vi "FipsAdjacent.vi"() -> (11 "Fips":i32[](array[numeric]))   [LabVIEW 2017] (continued)
MO\"\t29205\t\"Knox County, MO\"\t29103\n\"Shelby County, MO\"\t29205\t\"Lewis County, MO\"\t29111\n\"Shelby County, MO\"\t29205\t\"Macon County, MO\"\t29121\n\"Shelby County, MO\"\t29205\t\"Marion County, MO\"\t29127\n\"Shelby County, MO\"\t29205\t\"Monroe County, MO\"\t29137\n\"Shelby County, MO\"\t29205\t\"Shelby County, MO\"\t29205\n\"Stoddard County, MO\"\t29207\t\"Bollinger County, MO\"\t29017\n\"Stoddard County, MO\"\t29207\t\"Butler County, MO\"\t29023\n\"Stoddard County, MO\"\t29207\t\"Cape Girardeau County, MO\"\t29031\n\"Stoddard County, MO\"\t29207\t\"Dunklin County, MO\"\t29069\n\"Stoddard County, MO\"\t29207\t\"New Madrid County, MO\"\t29143\n\"Stoddard County, MO\"\t29207\t\"Scott County, MO\"\t29201\n\"Stoddard County, MO\"\t29207\t\"Stoddard County, MO\"\t29207\n\"Stoddard County, MO\"\t29207\t\"Wayne County, MO\"\t29223\n\"Stone County, MO\"\t29209\t\"Carroll County, AR\"\t05015\n\"Stone County, MO\"\t29209\t\"Barry County, MO\"\t29009\n\"Stone County, MO\"\t29209\t\"Christian County, MO\"\t29043\n\"Stone County, MO\"\t29209\t\"Lawrence County, MO\"\t29109\n\"Stone County, MO\"\t29209\t\"Stone County, MO\"\t29209\n\"Stone County, MO\"\t29209\t\"Taney County, MO\"\t29213\n\"Sullivan County, MO\"\t29211\t\"Adair County, MO\"\t29001\n\"Sullivan County, MO\"\t29211\t\"Grundy County, MO\"\t29079\n\"Sullivan County, MO\"\t29211\t\"Linn County, MO\"\t29115\n\"Sullivan County, MO\"\t29211\t\"Mercer County, MO\"\t29129\n\"Sullivan County, MO\"\t29211\t\"Putnam County, MO\"\t29171\n\"Sullivan County, MO\"\t29211\t\"Sullivan County, MO\"\t29211\n\"Taney County, MO\"\t29213\t\"Boone County, AR\"\t05009\n\"Taney County, MO\"\t29213\t\"Carroll County, AR\"\t05015\n\"Taney County, MO\"\t29213\t\"Marion County, AR\"\t05089\n\"Taney County, MO\"\t29213\t\"Christian County, MO\"\t29043\n\"Taney County, MO\"\t29213\t\"Douglas County, MO\"\t29067\n\"Taney County, MO\"\t29213\t\"Ozark County, MO\"\t29153\n\"Taney County, MO\"\t29213\t\"Stone County, MO\"\t29209\n\"Taney County, MO\"\t29213\t\"Taney County, MO\"\t29213\n\"Texas County, MO\"\t29215\t\"Dent County, MO\"\t29065\n\"Texas County, MO\"\t29215\t\"Douglas County, MO\"\t29067\n\"Texas County, MO\"\t29215\t\"Howell County, MO\"\t29091\n\"Texas County, MO\"\t29215\t\"Laclede County, MO\"\t29105\n\"Texas County, MO\"\t29215\t\"Phelps County, MO\"\t29161\n\"Texas County, MO\"\t29215\t\"Pulaski County, MO\"\t29169\n\"Texas County, MO\"\t29215\t\"Shannon County, MO\"\t29203\n\"Texas County, MO\"\t29215\t\"Texas County, MO\"\t29215\n\"Texas County, MO\"\t29215\t\"Wright County, MO\"\t29229\n\"Vernon County, MO\"\t29217\t\"Bourbon County, KS\"\t20011\n\"Vernon County, MO\"\t29217\t\"Crawford County, KS\"\t20037\n\"Vernon County, MO\"\t29217\t\"Linn County, KS\"\t20107\n\"Vernon County, MO\"\t29217\t\"Barton County, MO\"\t29011\n\"Vernon County, MO\"\t29217\t\"Bates County, MO\"\t29013\n\"Vernon County, MO\"\t29217\t\"Cedar County, MO\"\t29039\n\"Vernon County, MO\"\t29217\t\"St. Clair County, MO\"\t29185\n\"Vernon County, MO\"\t29217\t\"Vernon County, MO\"\t29217\n\"Warren County, MO\"\t29219\t\"Franklin County, MO\"\t29071\n\"Warren County, MO\"\t29219\t\"Gasconade County, MO\"\t29073\n\"Warren County, MO\"\t29219\t\"Lincoln County, MO\"\t29113\n\"Warren County, MO\"\t29219\t\"Montgomery County, MO\"\t29139\n\"Warren County, MO\"\t29219\t\"St. Charles County, MO\"\t29183\n\"Warren County, MO\"\t29219\t\"Warren County, MO\"\t29219\n\"Washington County, MO\"\t29221\t\"Crawford County, MO\"\t29055\n\"Washington County, MO\"\t29221\t\"Franklin County, MO\"\t29071\n\"Washington County, MO\"\t29221\t\"Iron County, MO\"\t29093\n\"Washington County, MO\"\t29221\t\"Jefferson County, MO\"\t29099\n\"Washington County, MO\"\t29221\t\"St. Francois County, MO\"\t29187\n\"Washington County, MO\"\t29221\t\"Washington County, MO\"\t29221\n\"Wayne County, MO\"\t29223\t\"Bollinger County, MO\"\t29017\n\"Wayne County, MO\"\t29223\t\"Butler County, MO\"\t29023\n\"Wayne County, MO\"\t29223\t\"Carter County, MO\"\t29035\n\"Wayne County, MO\"\t29223\t\"Iron County, MO\"\t29093\n\"Wayne County, MO\"\t29223\t\"Madison County, MO\"\t29123\n\"Wayne County, MO\"\t29223\t\"Reynolds County, MO\"\t29179\n\"Wayne County, MO\"\t29223\t\"Stoddard County, MO\"\t29207\n\"Wayne County, MO\"\t29223\t\"Wayne County, MO\"\t29223\n\"Webster County, MO\"\t29225\t\"Christian County, MO\"\t29043\n\"Webster County, MO\"\t29225\t\"Dallas County, MO\"\t29059\n\"Webster County, MO\"\t29225\t\"Douglas County, MO\"\t29067\n\"Webster County, MO\"\t29225\t\"Greene County, MO\"\t29077\n\"Webster County, MO\"\t29225\t\"Laclede County, MO\"\t29105\n\"Webster County, MO\"\t29225\t\"Webster County, MO\"\t29225\n\"Webster County, MO\"\t29225\t\"Wright County, MO\"\t29229\n\"Worth County, MO\"\t29227\t\"Ringgold County, IA\"\t19159\n\"Worth County, MO\"\t29227\t\"Taylor County, IA\"\t19173\n\"Worth County, MO\"\t29227\t\"Gentry County, MO\"\t29075\n\"Worth County, MO\"\t29227\t\"Harrison County, MO\"\t29081\n\"Worth County, MO\"\t29227\t\"Nodaway County, MO\"\t29147\n\"Worth County, MO\"\t29227\t\"Worth County, MO\"\t29227\n\"Wright County, MO\"\t29229\t\"Douglas County, MO\"\t29067\n\"Wright County, MO\"\t29229\t\"Laclede County, MO\"\t29105\n\"Wright County, MO\"\t29229\t\"Texas County, MO\"\t29215\n\"Wright County, MO\"\t29229\t\"Webster County, MO\"\t29225\n\"Wright County, MO\"\t29229\t\"Wright County, MO\"\t29229\n\"St. Louis city, MO\"\t29510\t\"Madison County, IL\"\t17119\n\"St. Louis city, MO\"\t29510\t\"St. Clair County, IL\"\t17163\n\"St. Louis city, MO\"\t29510\t\"St. Louis County, MO\"\t29189\n\"St. Louis city, MO\"\t29510\t\"St. Louis city, MO\"\t29510\n\"Beaverhead County, MT\"\t30001\t\"Clark County, ID\"\t16033\n\"Beaverhead County, MT\"\t30001\t\"Fremont County, ID\"\t16043\n\"Beaverhead County, MT\"\t30001\t\"Lemhi County, ID\"\t16059\n\"Beaverhead County, MT\"\t30001\t\"Beaverhead County, MT\"\t30001\n\"Beaverhead County, MT\"\t30001\t\"Deer Lodge County, MT\"\t30023\n\"Beaverhead County, MT\"\t30001\t\"Madison County, MT\"\t30057\n\"Beaverhead County, MT\"\t30001\t\"Ravalli County, MT\"\t30081\n\"Beaverhead County, MT\"\t30001\t\"Silver Bow County, MT\"\t30093\n\"Big Horn County, MT\"\t30003\t\"Big Horn County, MT\"\t30003\n\"Big Horn County, MT\"\t30003\t\"Carbon County, MT\"\t30009\n\"Big Horn County, MT\"\t30003\t\"Powder River County, MT\"\t30075\n\"Big Horn County, MT\"\t30003\t\"Rosebud County, MT\"\t30087\n\"Big Horn County, MT\"\t30003\t\"Treasure County, MT\"\t30103\n\"Big Horn County, MT\"\t30003\t\"Yellowstone County, MT\"\t30111\n\"Big Horn County, MT\"\t30003\t\"Big Horn County, WY\"\t56003\n\"Big Horn County, MT\"\t30003\t\"Sheridan County, WY\"\t56033\n\"Blaine County, MT\"\t30005\t\"Blaine County, MT\"\t30005\n\"Blaine County, MT\"\t30005\t\"Chouteau County, MT\"\t30015\n\"Blaine County, MT\"\t30005\t\"Fergus County, MT\"\t30027\n\"Blaine County, MT\"\t30005\t\"Hill County, MT\"\t30041\n\"Blaine County, MT\"\t30005\t\"Phillips County, MT\"\t30071\n\"Broadwater County, MT\"\t30007\t\"Broadwater County, MT\"\t30007\n\"Broadwater County, MT\"\t30007\t\"Gallatin County, MT\"\t30031\n\"Broadwater County, MT\"\t30007\t\"Jefferson County, MT\"\t30043\n\"Broadwater County, MT\"\t30007\t\"Lewis and Clark County, MT\"\t30049\n\"Broadwater County, MT\"\t30007\t\"Meagher County, MT\"\t30059\n\"Carbon County, MT\"\t30009\t\"Big Horn County, MT\"\t30003\n\"Carbon County, MT\"\t30009\t\"Carbon County, MT\"\t30009\n\"Carbon County, MT\"\t30009\t\"Park County, MT\"\t30067\n\"Carbon County, MT\"\t30009\t\"Stillwater County, MT\"\t30095\n\"Carbon County, MT\"\t30009\t\"Yellowstone County, MT\"\t30111\n\"Carbon County, MT\"\t30009\t\"Big Horn County, WY\"\t56003\n\"Carbon County, MT\"\t30009\t\"Park County, WY\"\t56029\n\"Carter County, MT\"\t30011\t\"Carter County, MT\"\t30011\n\"Carter County, MT\"\t30011\t\"Custer County, MT\"\t30017\n\"Carter County, MT\"\t30011\t\"Fallon County, MT\"\t30025\n\"Carter County, MT\"\t30011\t\"Powder River County, MT\"\t30075\n\"Carter County, MT\"\t30011\t\"Butte County, SD\"\t46019\n\"Carter County, MT\"\t30011\t\"Harding County, SD\"\t46063\n\"Carter County, MT\"\t30011\t\"Crook County, WY\"\t56011\n\"Cascade County, MT\"\t30013\t\"Cascade County, MT\"\t30013\n\"Cascade County, MT\"\t30013\t\"Chouteau County, MT\"\t30015\n\"Cascade County, MT\"\t30013\t\"Judith Basin County, MT\"\t30045\n\"Cascade County, MT\"\t30013\t\"Lewis and Clark County, MT\"\t30049\n\"Cascade County, MT\"\t30013\t\"Meagher County, MT\"\t30059\n\"Cascade County, MT\"\t30013\t\"Teton County, MT\"\t30099\n\"Chouteau County, MT\"\t30015\t\"Blaine County, MT\"\t30005\n\"Chouteau County, MT\"\t30015\t\"Cascade County, MT\"\t30013\n\"Chouteau County, MT\"\t30015\t\"Chouteau County, MT\"\t30015\n\"Chouteau County, MT\"\t30015\t\"Fergus County, MT\"\t30027\n\"Chouteau County, MT\"\t30015\t\"Hill County, MT\"\t30041\n\"Chouteau County, MT\"\t30015\t\"Judith Basin County, MT\"\t30045\n\"Chouteau County, MT\"\t30015\t\"Liberty County, MT\"\t30051\n\"Chouteau County, MT\"\t30015\t\"Pondera County, MT\"\t30073\n\"Chouteau County, MT\"\t30015\t\"Teton County, MT\"\t30099\n\"Custer County, MT\"\t30017\t\"Carter County, MT\"\t30011\n\"Custer County, MT\"\t30017\t\"Custer County, MT\"\t30017\n\"Custer County, MT\"\t30017\t\"Fallon County, MT\"\t30025\n\"Custer County, MT\"\t30017\t\"Garfield County, MT\"\t30033\n\"Custer County, MT\"\t30017\t\"Powder River County, MT\"\t30075\n\"Custer County, MT\"\t30017\t\"Prairie County, MT\"\t30079\n\"Custer County, MT\"\t30017\t\"Rosebud County, MT\"\t30087\n\"Daniels County, MT\"\t30019\t\"Daniels County, MT\"\t30019\n\"Daniels County, MT\"\t30019\t\"Roosevelt County, MT\"\t30085\n\"Daniels County, MT\"\t30019\t\"Sheridan County, MT\"\t30091\n\"Daniels County, MT\"\t30019\t\"Valley County, MT\"\t30105\n\"Dawson County, MT\"\t30021\t\"Dawson County, MT\"\t30021\n\"Dawson County, MT\"\t30021\t\"McCone County, MT\"\t30055\n\"Dawson County, MT\"\t30021\t\"Prairie County, MT\"\t30079\n\"Dawson County, MT\"\t30021\t\"Richland County, MT\"\t30083\n\"Dawson County, MT\"\t30021\t\"Wibaux County, MT\"\t30109\n\"Deer Lodge County, MT\"\t30023\t\"Beaverhead County, MT\"\t30001\n\"Deer Lodge County, MT\"\t30023\t\"Deer Lodge County, MT\"\t30023\n\"Deer Lodge County, MT\"\t30023\t\"Granite County, MT\"\t30039\n\"Deer Lodge County, MT\"\t30023\t\"Jefferson County, MT\"\t30043\n\"Deer Lodge County, MT\"\t30023\t\"Powell County, MT\"\t30077\n\"Deer Lodge County, MT\"\t30023\t\"Ravalli County, MT\"\t30081\n\"Deer Lodge County, MT\"\t30023\t\"Silver Bow County, MT\"\t30093\n\"Fallon County, MT\"\t30025\t\"Carter County, MT\"\t30011\n\"Fallon County, MT\"\t30025\t\"Custer County, MT\"\t30017\n\"Fallon County, MT\"\t30025\t\"Fallon County, MT\"\t30025\n\"Fallon County, MT\"\t30025\t\"Prairie County, MT\"\t30079\n\"Fallon County, MT\"\t30025\t\"Wibaux County, MT\"\t30109\n\"Fallon County, MT\"\t30025\t\"Bowman County, ND\"\t38011\n\"Fallon County, MT\"\t30025\t\"Golden Valley County, ND\"\t38033\n\"Fallon County, MT\"\t30025\t\"Slope County, ND\"\t38087\n\"Fallon County, MT\"\t30025\t\"Harding County, SD\"\t46063\n\"Fergus County, MT\"\t30027\t\"Blaine County, MT\"\t30005\n\"Fergus County, MT\"\t30027\t\"Chouteau County, MT\"\t30015\n\"Fergus County, MT\"\t30027\t\"Fergus County, MT\"\t30027\n\"Fergus County, MT\"\t30027\t\"Golden Valley County, MT\"\t30037\n\"Fergus County, MT\"\t30027\t\"Judith Basin County, MT\"\t30045\n\"Fergus County, MT\"\t30027\t\"Musselshell County, MT\"\t30065\n\"Fergus County, MT\"\t30027\t\"Petroleum County, MT\"\t30069\n\"Fergus County, MT\"\t30027\t\"Phillips County, MT\"\t30071\n\"Fergus County, MT\"\t30027\t\"Wheatland County, MT\"\t30107\n\"Flathead County, MT\"\t30029\t\"Flathead County, MT\"\t30029\n\"Flathead County, MT\"\t30029\t\"Glacier County, MT\"\t30035\n\"Flathead County, MT\"\t30029\t\"Lake County, MT\"\t30047\n\"Flathead County, MT\"\t30029\t\"Lewis and Clark County, MT\"\t30049\n\"Flathead County, MT\"\t30029\t\"Lincoln County, MT\"\t30053\n\"Flathead County, MT\"\t30029\t\"Missoula County, MT\"\t30063\n\"Flathead County, MT\"\t30029\t\"Pondera County, MT\"\t30073\n\"Flathead County, MT\"\t30029\t\"Powell County, MT\"\t30077\n\"Flathead County, MT\"\t30029\t\"Sanders County, MT\"\t30089\n\"Flathead County, MT\"\t30029\t\"Teton County, MT\"\t30099\n\"Gallatin County, MT\"\t30031\t\"Fremont County, ID\"\t16043\n\"Gallatin County, MT\"\t30031\t\"Broadwater County, MT\"\t30007\n\"Gallatin County, MT\"\t30031\t\"Gallatin County, MT\"\t30031\n\"Gallatin County, MT\"\t30031\t\"Jefferson County, MT\"\t30043\n\"Gallatin County, MT\"\t30031\t\"Madison County, MT\"\t30057\n\"Gallatin County, MT\"\t30031\t\"Meagher County, MT\"\t30059\n\"Gallatin County, MT\"\t30031\t\"Park County, MT\"\t30067\n\"Gallatin County, MT\"\t30031\t\"Park County, WY\"\t56029\n\"Gallatin County, MT\"\t30031\t\"Teton County, WY\"\t56039\n\"Garfield County, MT\"\t30033\t\"Custer County, MT\"\t30017\n\"Garfield County, MT\"\t30033\t\"Garfield County, MT\"\t30033\n\"Garfield County, MT\"\t30033\t\"McCone County, MT\"\t30055\n\"Garfield County, MT\"\t30033\t\"Petroleum County, MT\"\t30069\n\"Garfield County, MT\"\t30033\t\"Phillips County, MT\"\t30071\n\"Garfield County, MT\"\t30033\t\"Prairie County, MT\"\t30079\n\"Garfield County, MT\"\t30033\t\"Rosebud County, MT\"\t30087\n\"Garfield County, MT\"\t30033\t\"Valley County, MT\"\t30105\n\"Glacier County, MT\"\t30035\t\"Flathead County, MT\"\t30029\n\"Glacier County, MT\"\t30035\t\"Glacier County, MT\"\t30035\n\"Glacier County, MT\"\t30035\t\"Pondera County, MT\"\t30073\n\"Glacier County, MT\"\t30035\t\"Toole County, MT\"\t30101\n\"Golden Valley County, MT\"\t30037\t\"Fergus County, MT\"\t30027\n\"Golden Valley County, MT\"\t30037\t\"Golden Valley County, MT\"\t30037\n\"Golden Valley County, MT\"\t30037\t\"Musselshell County, MT\"\t30065\n\"Golden Valley County, MT\"\t30037\t\"Stillwater County, MT\"\t30095\n\"Golden Valley County, MT\"\t30037\t\"Sweet Grass County, MT\"\t30097\n\"Golden Valley County, MT\"\t30037\t\"Wheatland County, MT\"\t30107\n\"Golden Valley County, MT\"\t30037\t\"Yellowstone County, MT\"\t30111\n\"Granite County, MT\"\t30039\t\"Deer Lodge County, MT\"\t30023\n\"Granite County, MT\"\t30039\t\"Granite County, MT\"\t30039\n\"Granite County, MT\"\t30039\t\"Missoula County, MT\"\t30063\n\"Granite County, MT\"\t30039\t\"Powell County, MT\"\t30077\n\"Granite County, MT\"\t30039\t\"Ravalli County, MT\"\t30081\n\"Hill County, MT\"\t30041\t\"Blaine County, MT\"\t30005\n\"Hill County, MT\"\t30041\t\"Chouteau County, MT\"\t30015\n\"Hill County, MT\"\t30041\t\"Hill County, MT\"\t30041\n\"Hill County, MT\"\t30041\t\"Liberty County, MT\"\t30051\n\"Jefferson County, MT\"\t30043\t\"Broadwater County, MT\"\t30007\n\"Jefferson County, MT\"\t30043\t\"Deer Lodge County, MT\"\t30023\n\"Jefferson County, MT\"\t30043\t\"Gallatin County, MT\"\t30031\n\"Jefferson County, MT\"\t30043\t\"Jefferson County, MT\"\t30043\n\"Jefferson County, MT\"\t30043\t\"Lewis and Clark County, MT\"\t30049\n\"Jefferson County, MT\"\t30043\t\"Madison County, MT\"\t30057\n\"Jefferson County, MT\"\t30043\t\"Powell County, MT\"\t30077\n\"Jefferson County, MT\"\t30043\t\"Silver Bow County, MT\"\t30093\n\"Judith Basin County, MT\"\t30045\t\"Cascade County, MT\"\t30013\n\"Judith Basin County, MT\"\t30045\t\"Chouteau County, MT\"\t30015\n\"Judith Basin County, MT\"\t30045\t\"Fergus County, MT\"\t30027\n\"Judith Basin County, MT\"\t30045\t\"Judith Basin County, MT\"\t30045\n\"Judith Basin County, MT\"\t30045\t\"Meagher County, MT\"\t30059\n\"Judith Basin County, MT\"\t30045\t\"Wheatland County, MT\"\t30107\n\"Lake County, MT\"\t30047\t\"Flathead County, MT\"\t30029\n\"Lake County, MT\"\t30047\t\"Lake County, MT\"\t30047\n\"Lake County, MT\"\t30047\t\"Missoula County, MT\"\t30063\n\"Lake County, MT\"\t30047\t\"Sanders County, MT\"\t30089\n\"Lewis and Clark County, MT\"\t30049\t\"Broadwater County, MT\"\t30007\n\"Lewis and Clark County, MT\"\t30049\t\"Cascade County, MT\"\t30013\n\"Lewis and Clark County, MT\"\t30049\t\"Flathead County, MT\"\t30029\n\"Lewis and Clark County, MT\"\t30049\t\"Jefferson County, MT\"\t30043\n\"Lewis and Clark County, MT\"\t30049\t\"Lewis and Clark County, MT\"\t30049\n\"Lewis and Clark County, MT\"\t30049\t\"Meagher County, MT\"\t30059\n\"Lewis and Clark County, MT\"\t30049\t\"Powell County, MT\"\t30077\n\"Lewis and Clark County, MT\"\t30049\t\"Teton County, MT\"\t30099\n\"Liberty County, MT\"\t30051\t\"Chouteau County, MT\"\t30015\n\"Liberty County, MT\"\t30051\t\"Hill County, MT\"\t30041\n\"Liberty County, MT\"\t30051\t\"Liberty County, MT\"\t30051\n\"Liberty County, MT\"\t30051\t\"Pondera County, MT\"\t30073\n\"Liberty County, MT\"\t30051\t\"Toole County, MT\"\t30101\n\"Lincoln County, MT\"\t30053\t\"Bonner County, ID\"\t16017\n\"Lincoln County, MT\"\t30053\t\"Boundary County, ID\"\t16021\n\"Lincoln County, MT\"\t30053\t\"Flathead County, MT\"\t30029\n\"Lincoln County, MT\"\t30053\t\"Lincoln County, MT\"\t30053\n\"Lincoln County, MT\"\t30053\t\"Sanders County, MT\"\t30089\n\"McCone County, MT\"\t30055\t\"Dawson County, MT\"\t30021\n\"McCone County, MT\"\t30055\t\"Garfield County, MT\"\t30033\n\"McCone County, MT\"\t30055\t\"McCone County, MT\"\t30055\n\"McCone County, MT\"\t30055\t\"Prairie County, MT\"\t30079\n\"McCone County, MT\"\t30055\t\"Richland County, MT\"\t30083\n\"McCone County, MT\"\t30055\t\"Roosevelt County, MT\"\t30085\n\"McCone County, MT\"\t30055\t\"Valley County, MT\"\t30105\n\"Madison County, MT\"\t30057\t\"Fremont County, ID\"\t16043\n\"Madison County, MT\"\t30057\t\"Beaverhead County, MT\"\t30001\n\"Madison County, MT\"\t30057\t\"Gallatin County, MT\"\t30031\n\"Madison County, MT\"\t30057\t\"Jefferson County, MT\"\t30043\n\"Madison County, MT\"\t30057\t\"Madison County, MT\"\t30057\n\"Madison County, MT\"\t30057\t\"Silver Bow County, MT\"\t30093\n\"Meagher County, MT\"\t30059\t\"Broadwater County, MT\"\t30007\n\"Meagher County, MT\"\t30059\t\"Cascade County, MT\"\t30013\n\"Meagher County, MT\"\t30059\t\"Gallatin County, MT\"\t30031\n\"Meagher County, MT\"\t30059\t\"Judith Basin County, MT\"\t30045\n\"Meagher County, MT\"\t30059\t\"Lewis and Clark County, MT\"\t30049\n\"Meagher County, MT\"\t30059\t\"Meagher County, MT\"\t30059\n\"Meagher County, MT\"\t30059\t\"Park County, MT\"\t30067\n\"Meagher County, MT\"\t30059\t\"Sweet Grass County, MT\"\t30097\n\"Meagher County, MT\"\t30059\t\"Wheatland County, MT\"\t30107\n\"Mineral County, MT\"\t30061\t\"Clearwater County, ID\"\t16035\n\"Mineral County, MT\"\t30061\t\"Shoshone County, ID\"\t16079\n\"Mineral County, MT\"\t30061\t\"Mineral County, MT\"\t30061\n\"Mineral County, MT\"\t30061\t\"Missoula County, MT\"\t30063\n\"Mineral County, MT\"\t30061\t\"Sanders County, MT\"\t30089\n\"Missoula County, MT\"\t30063\t\"Clearwater County, ID\"\t16035\n\"Missoula County, MT\"\t30063\t\"Idaho County, ID\"\t16049\n\"Missoula County, MT\"\t30063\t\"Flathead County, MT\"\t30029\n\"Missoula County, MT\"\t30063\t\"Granite County, MT\"\t30039\n\"Missoula County, MT\"\t30063\t\"Lake County, MT\"\t30047\n\"Missoula County, MT\"\t30063\t\"Mineral County, MT\"\t30061\n\"Missoula County, MT\"\t30063\t\"Missoula County, MT\"\t30063\n\"Missoula County, MT\"\t30063\t\"Powell County, MT\"\t30077\n\"Missoula County, MT\"\t30063\t\"Ravalli County, MT\"\t30081\n\"Missoula County, MT\"\t30063\t\"Sanders County, MT\"\t30089\n\"Musselshell County, MT\"\t30065\t\"Fergus County, MT\"\t30027\n\"Musselshell County, MT\"\t30065\t\"Golden Valley County, MT\"\t30037\n\"Musselshell County, MT\"\t30065\t\"Musselshell County, MT\"\t30065\n\"Musselshell County, MT\"\t30065\t\"Petroleum County, MT\"\t30069\n\"Musselshell County, MT\"\t30065\t\"Rosebud County, MT\"\t30087\n\"Musselshell County, MT\"\t30065\t\"Yellowstone County, MT\"\t30111\n\"Park County, MT\"\t30067\t\"Carbon County, MT\"\t30009\n\"Park County, MT\"\t30067\t\"Gallatin County, MT\"\t30031\n\"Park County, MT\"\t30067\t\"Meagher County, MT\"\t30059\n\"Park County, MT\"\t30067\t\"Park County, MT\"\t30067\n\"Park County, MT\"\t30067\t\"Stillwater County, MT\"\t30095\n\"Park County, MT\"\t30067\t\"Sweet Grass County, MT\"\t30097\n\"Park County, MT\"\t30067\t\"Park County, WY\"\t56029\n\"Petroleum County, MT\"\t30069\t\"Fergus County, MT\"\t30027\n\"Petroleum County, MT\"\t30069\t\"Garfield County, MT\"\t30033\n\"Petroleum County, MT\"\t30069\t\"Musselshell County, MT\"\t30065\n\"Petroleum County, MT\"\t30069\t\"Petroleum County, MT\"\t30069\n\"Petroleum County, MT\"\t30069\t\"Phillips County, MT\"\t30071\n\"Petroleum County, MT\"\t30069\t\"Rosebud County, MT\"\t30087\n\"Phillips County, MT\"\t30071\t\"Blaine County, MT\"\t30005\n\"Phillips County, MT\"\t30071\t\"Fergus County, MT\"\t30027\n\"Phillips County, MT\"\t30071\t\"Garfield County, MT\"\t30033\n\"Phillips County, MT\"\t30071\t\"Petroleum County, MT\"\t30069\n\"Phillips County, MT\"\t30071\t\"Phillips County, MT\"\t30071\n\"Phillips County, MT\"\t30071\t\"Valley County, MT\"\t30105\n\"Pondera County, MT\"\t30073\t\"Chouteau County, MT\"\t30015\n\"Pondera County, MT\"\t30073\t\"Flathead County, MT\"\t30029\n\"Pondera County, MT\"\t30073\t\"Glacier County, MT\"\t30035\n\"Pondera County, MT\"\t30073\t\"Liberty County, MT\"\t30051\n\"Pondera County, MT\"\t30073\t\"Pondera County, MT\"\t30073\n\"Pondera County, MT\"\t30073\t\"Teton County, MT\"\t30099\n\"Pondera County, MT\"\t30073\t\"Toole County, MT\"\t30101\n\"Powder River County, MT\"\t30075\t\"Big Horn County, MT\"\t30003\n\"Powder River County, MT\"\t30075\t\"Carter County, MT\"\t30011\n\"Powder River County, MT\"\t30075\t\"Custer County, MT\"\t30017\n\"Powder River County, MT\"\t30075\t\"Powder River County, MT\"\t30075\n\"Powder River County, MT\"\t30075\t\"Rosebud County, MT\"\t30087\n\"Powder River County, MT\"\t30075\t\"Campbell County, WY\"\t56005\n\"Powder River County, MT\"\t30075\t\"Crook County, WY\"\t56011\n\"Powder River County, MT\"\t30075\t\"Sheridan County, WY\"\t56033\n\"Powell County, MT\"\t30077\t\"Deer Lodge County, MT\"\t30023\n\"Powell County, MT\"\t30077\t\"Flathead County, MT\"\t30029\n\"Powell County, MT\"\t30077\t\"Granite County, MT\"\t30039\n\"Powell County, MT\"\t30077\t\"Jefferson County, MT\"\t30043\n\"Powell County, MT\"\t30077\t\"Lewis and Clark County, MT\"\t30049\n\"Powell County, MT\"\t30077\t\"Missoula County, MT\"\t30063\n\"Powell County, MT\"\t30077\t\"Powell County, MT\"\t30077\n\"Prairie County, MT\"\t30079\t\"Custer County, MT\"\t30017\n\"Prairie County, MT\"\t30079\t\"Dawson County, MT\"\t30021\n\"Prairie County, MT\"\t30079\t\"Fallon County, MT\"\t30025\n\"Prairie County, MT\"\t30079\t\"Garfield County, MT\"\t30033\n\"Prairie County, MT\"\t30079\t\"McCone County, MT\"\t30055\n\"Prairie County, MT\"\t30079\t\"Prairie County, MT\"\t30079\n\"Prairie County, MT\"\t30079\t\"Wibaux County, MT\"\t30109\n\"Ravalli County, MT\"\t30081\t\"Idaho County, ID\"\t16049\n\"Ravalli County, MT\"\t30081\t\"Lemhi County, ID\"\t16059\n\"Ravalli County, MT\"\t30081\t\"Beaverhead County, MT\"\t30001\n\"Ravalli County, MT\"\t30081\t\"Deer Lodge County, MT\"\t30023\n\"Ravalli County, MT\"\t30081\t\"Granite County, MT\"\t30039\n\"Ravalli County, MT\"\t30081\t\"Missoula County, MT\"\t30063\n\"Ravalli County, MT\"\t30081\t\"Ravalli County, MT\"\t30081\n\"Richland County, MT\"\t30083\t\"Dawson County, MT\"\t30021\n\"Richland County, MT\"\t30083\t\"McCone County, MT\"\t30055\n\"Richland County, MT\"\t30083\t\"Richland County, MT\"\t30083\n\"Richland County, MT\"\t30083\t\"Roosevelt County, MT\"\t30085\n\"Richland County, MT\"\t30083\t\"Wibaux County, MT\"\t30109\n\"Richland County, MT\"\t30083\t\"McKenzie County, ND\"\t38053\n\"Richland County, MT\"\t30083\t\"Williams County, ND\"\t38105\n\"Roosevelt County, MT\"\t30085\t\"Daniels County, MT\"\t30019\n\"Roosevelt County, MT\"\t30085\t\"McCone County, MT\"\t30055\n\"Roosevelt County, MT\"\t30085\t\"Richland County, MT\"\t30083\n\"Roosevelt County, MT\"\t30085\t\"Roosevelt County, MT\"\t30085\n\"Roosevelt County, MT\"\t30085\t\"Sheridan County, MT\"\t30091\n\"Roosevelt County, MT\"\t30085\t\"Valley County, MT\"\t30105\n\"Roosevelt County, MT\"\t30085\t\"McKenzie County, ND\"\t38053\n\"Roosevelt County, MT\"\t30085\t\"Williams County, ND\"\t38105\n\"Rosebud County, MT\"\t30087\t\"Big Horn County, MT\"\t30003\n\"Rosebud County, MT\"\t30087\t\"Custer County, MT\"\t30017\n\"Rosebud County, MT\"\t30087\t\"Garfield County, MT\"\t30033\n\"Rosebud County, MT\"\t30087\t\"Musselshell County, MT\"\t30065\n\"Rosebud County, MT\"\t30087\t\"Petroleum County, MT\"\t30069\n\"Rosebud County, MT\"\t30087\t\"Powder River County, MT\"\t30075\n\"Rosebud County, MT\"\t30087\t\"Rosebud County, MT\"\t30087\n\"Rosebud County, MT\"\t30087\t\"Treasure County, MT\"\t30103\n\"Rosebud County, MT\"\t30087\t\"Yellowstone County, MT\"\t30111\n\"Sanders County, MT\"\t30089\t\"Bonner County, ID\"\t16017\n\"Sanders County, MT\"\t30089\t\"Shoshone County, ID\"\t16079\n\"Sanders County, MT\"\t30089\t\"Flathead County, MT\"\t30029\n\"Sanders County, MT\"\t30089\t\"Lake County, MT\"\t30047\n\"Sanders County, MT\"\t30089\t\"Lincoln County, MT\"\t30053\n\"Sanders County, MT\"\t30089\t\"Mineral County, MT\"\t30061\n\"Sanders County, MT\"\t30089\t\"Missoula County, MT\"\t30063\n\"Sanders County, MT\"\t30089\t\"Sanders County, MT\"\t30089\n\"Sheridan County, MT\"\t30091\t\"Daniels County, MT\"\t30019\n\"Sheridan County, MT\"\t30091\t\"Roosevelt County, MT\"\t30085\n\"Sheridan County, MT\"\t30091\t\"Sheridan County, MT\"\t30091\n\"Sheridan County, MT\"\t30091\t\"Divide County, ND\"\t38023\n\"Sheridan County, MT\"\t30091\t\"Williams County, ND\"\t38105\n\"Silver Bow County, MT\"\t30093\t\"Beaverhead County, MT\"\t30001\n\"Silver Bow County, MT\"\t30093\t\"Deer Lodge County, MT\"\t30023\n\"Silver Bow County, MT\"\t30093\t\"Jefferson County, MT\"\t30043\n\"Silver Bow County, MT\"\t30093\t\"Madison County, MT\"\t30057\n\"Silver Bow County, MT\"\t30093\t\"Silver Bow County, MT\"\t30093\n\"Stillwater County, MT\"\t30095\t\"Carbon County, MT\"\t30009\n\"Stillwater County, MT\"\t30095\t\"Golden Valley County, MT\"\t30037\n\"Stillwater County, MT\"\t30095\t\"Park County, MT\"\t30067\n\"Stillwater County, MT\"\t30095\t\"Stillwater County, MT\"\t30095\n\"Stillwater County, MT\"\t30095\t\"Sweet Grass County, MT\"\t30097\n\"Stillwater County, MT\"\t30095\t\"Yellowstone County, MT\"\t30111\n\"Sweet Grass County, MT\"\t30097\t\"Golden Valley County, MT\"\t30037\n\"Sweet Grass County, MT\"\t30097\t\"Meagher County, MT\"\t30059\n\"Sweet Grass County, MT\"\t30097\t\"Park County, MT\"\t30067\n\"Sweet Grass County, MT\"\t30097\t\"Stillwater County, MT\"\t30095\n\"Sweet Grass County, MT\"\t30097\t\"Sweet Grass County, MT\"\t30097\n\"Sweet Grass County, MT\"\t30097\t\"Wheatland County, MT\"\t30107\n\"Teton County, MT\"\t30099\t\"Cascade County, MT\"\t30013\n\"Teton County, MT\"\t30099\t\"Chouteau County, MT\"\t30015\n\"Teton County, MT\"\t30099\t\"Flathead County, MT\"\t30029\n\"Teton County, MT\"\t30099\t\"Lewis and Clark County, MT\"\t30049\n\"Teton County, MT\"\t30099\t\"Pondera County, MT\"\t30073\n\"Teton County, MT\"\t30099\t\"Teton County, MT\"\t30099\n\"Toole County, MT\"\t30101\t\"Glacier County, MT\"\t30035\n\"Toole County, MT\"\t30101\t\"Liberty County, MT\"\t30051\n\"Toole County, MT\"\t30101\t\"Pondera County, MT\"\t30073\n\"Toole County, MT\"\t30101\t\"Toole County, MT\"\t30101\n\"Treasure County, MT\"\t30103\t\"Big Horn County, MT\"\t30003\n\"Treasure County, MT\"\t30103\t\"Rosebud County, MT\"\t30087\n\"Treasure County, MT\"\t30103\t\"Treasure County, MT\"\t30103\n\"Treasure County, MT\"\t30103\t\"Yellowstone County, MT\"\t30111\n\"Valley County, MT\"\t30105\t\"Daniels County, MT\"\t30019\n\"Valley County, MT\"\t30105\t\"Garfield County, MT\"\t30033\n\"Valley County, MT\"\t30105\t\"McCone County, MT\"\t30055\n\"Valley County, MT\"\t30105\t\"Phillips County, MT\"\t30071\n\"Valley County, MT\"\t30105\t\"Roosevelt County, MT\"\t30085\n\"Valley County, MT\"\t30105\t\"Valley County, MT\"\t30105\n\"Wheatland County, MT\"\t30107\t\"Fergus County, MT\"\t30027\n\"Wheatland County, MT\"\t30107\t\"Golden Valley County, MT\"\t30037\n\"Wheatland County, MT\"\t30107\t\"Judith Basin County, MT\"\t30045\n\"Wheatland County, MT\"\t30107\t\"Meagher County, MT\"\t30059\n\"Wheatland County, MT\"\t30107\t\"Sweet Grass County, MT\"\t30097\n\"Wheatland County, MT\"\t30107\t\"Wheatland County, MT\"\t30107\n\"Wibaux County, MT\"\t30109\t\"Dawson County, MT\"\t30021\n\"Wibaux County, MT\"\t30109\t\"Fallon County, MT\"\t30025\n\"Wibaux County, MT\"\t30109\t\"Prairie County, MT\"\t30079\n\"Wibaux County, MT\"\t30109\t\"Richland County, MT\"\t30083\n\"Wibaux County, MT\"\t30109\t\"Wibaux County, MT\"\t30109\n\"Wibaux County, MT\"\t30109\t\"Golden Valley County, ND\"\t38033\n\"Wibaux County, MT\"\t30109\t\"McKenzie County, ND\"\t38053\n\"Yellowstone County, MT\"\t30111\t\"Big Horn County, MT\"\t30003\n\"Yellowstone County, MT\"\t30111\t\"Carbon County, MT\"\t30009\n\"Yellowstone County, MT\"\t30111\t\"Golden Valley County, MT\"\t30037\n\"Yellowstone County, MT\"\t30111\t\"Musselshell County, MT\"\t30065\n\"Yellowstone County, MT\"\t30111\t\"Rosebud County, MT\"\t30087\n\"Yellowstone County, MT\"\t30111\t\"Stillwater County, MT\"\t30095\n\"Yellowstone County, MT\"\t30111\t\"Treasure County, MT\"\t30103\n\"Yellowstone County, MT\"\t30111\t\"Yellowstone County, MT\"\t30111\n\"Adams County, NE\"\t31001\t\"Adams County, NE\"\t31001\n\"Adams County, NE\"\t31001\t\"Buffalo County, NE\"\t31019\n\"Adams County, NE\"\t31001\t\"Clay County, NE\"\t31035\n\"Adams County, NE\"\t31001\t\"Hall County, NE\"\t31079\n\"Adams County, NE\"\t31001\t\"Hamilton County, NE\"\t31081\n\"Adams County, NE\"\t31001\t\"Kearney County, NE\"\t31099\n\"Adams County, NE\"\t31001\t\"Webster County, NE\"\t31181\n\"Antelope County, NE\"\t31003\t\"Antelope County, NE\"\t31003\n\"Antelope County, NE\"\t31003\t\"Boone County, NE\"\t31011\n\"Antelope County, NE\"\t31003\t\"Holt County, NE\"\t31089\n\"Antelope County, NE\"\t31003\t\"Knox County, NE\"\t31107\n\"Antelope County, NE\"\t31003\t\"Madison County, NE\"\t31119\n\"Antelope County, NE\"\t31003\t\"Pierce County, NE\"\t31139\n\"Antelope County, NE\"\t31003\t\"Wheeler County, NE\"\t31183\n\"Arthur County, NE\"\t31005\t\"Arthur County, NE\"\t31005\n\"Arthur County, NE\"\t31005\t\"Garden County, NE\"\t31069\n\"Arthur County, NE\"\t31005\t\"Grant County, NE\"\t31075\n\"Arthur County, NE\"\t31005\t\"Hooker County, NE\"\t31091\n\"Arthur County, NE\"\t31005\t\"Keith County, NE\"\t31101\n\"Arthur County, NE\"\t31005\t\"McPherson County, NE\"\t31117\n\"Banner County, NE\"\t31007\t\"Banner County, NE\"\t31007\n\"Banner County, NE\"\t31007\t\"Cheyenne County, NE\"\t31033\n\"Banner County, NE\"\t31007\t\"Kimball County, NE\"\t31105\n\"Banner County, NE\"\t31007\t\"Morrill County, NE\"\t31123\n\"Banner County, NE\"\t31007\t\"Scotts Bluff County, NE\"\t31157\n\"Banner County, NE\"\t31007\t\"Goshen County, WY\"\t56015\n\"Banner County, NE\"\t31007\t\"Laramie County, WY\"\t56021\n\"Blaine County, NE\"\t31009\t\"Blaine County, NE\"\t31009\n\"Blaine County, NE\"\t31009\t\"Brown County, NE\"\t31017\n\"Blaine County, NE\"\t31009\t\"Cherry County, NE\"\t31031\n\"Blaine County, NE\"\t31009\t\"Custer County, NE\"\t31041\n\"Blaine County, NE\"\t31009\t\"Logan County, NE\"\t31113\n\"Blaine County, NE\"\t31009\t\"Loup County, NE\"\t31115\n\"Blaine County, NE\"\t31009\t\"Thomas County, NE\"\t31171\n\"Boone County, NE\"\t31011\t\"Antelope County, NE\"\t31003\n\"Boone County, NE\"\t31011\t\"Boone County, NE\"\t31011\n\"Boone County, NE\"\t31011\t\"Greeley County, NE\"\t31077\n\"Boone County, NE\"\t31011\t\"Madison County, NE\"\t31119\n\"Boone County, NE\"\t31011\t\"Nance County, NE\"\t31125\n\"Boone County, NE\"\t31011\t\"Platte County, NE\"\t31141\n\"Boone County, NE\"\t31011\t\"Wheeler County, NE\"\t31183\n\"Box Butte County, NE\"\t31013\t\"Box Butte County, NE\"\t31013\n\"Box Butte County, NE\"\t31013\t\"Dawes County, NE\"\t31045\n\"Box Butte County, NE\"\t31013\t\"Morrill County, NE\"\t31123\n\"Box Butte County, NE\"\t31013\t\"Scotts Bluff County, NE\"\t31157\n\"Box Butte County, NE\"\t31013\t\"Sheridan County, NE\"\t31161\n\"Box Butte County, NE\"\t31013\t\"Sioux County, NE\"\t31165\n\"Boyd County, NE\"\t31015\t\"Boyd County, NE\"\t31015\n\"Boyd County, NE\"\t31015\t\"Holt County, NE\"\t31089\n\"Boyd County, NE\"\t31015\t\"Keya Paha County, NE\"\t31103\n\"Boyd County, NE\"\t31015\t\"Knox County, NE\"\t31107\n\"Boyd County, NE\"\t31015\t\"Rock County, NE\"\t31149\n\"Boyd County, NE\"\t31015\t\"Charles Mix County, SD\"\t46023\n\"Boyd County, NE\"\t31015\t\"Gregory County, SD\"\t46053\n\"Brown County, NE\"\t31017\t\"Blaine County, NE\"\t31009\n\"Brown County, NE\"\t31017\t\"Brown County, NE\"\t31017\n\"Brown County, NE\"\t31017\t\"Cherry County, NE\"\t31031\n\"Brown County, NE\"\t31017\t\"Keya Paha County, NE\"\t31103\n\"Brown County, NE\"\t31017\t\"Loup County, NE\"\t31115\n\"Brown County, NE\"\t31017\t\"Rock County, NE\"\t31149\n\"Buffalo County, NE\"\t31019\t\"Adams County, NE\"\t31001\n\"Buffalo County, NE\"\t31019\t\"Buffalo County, NE\"\t31019\n\"Buffalo County, NE\"\t31019\t\"Custer County, NE\"\t31041\n\"Buffalo County, NE\"\t31019\t\"Dawson County, NE\"\t31047\n\"Buffalo County, NE\"\t31019\t\"Hall County, NE\"\t31079\n\"Buffalo County, NE\"\t31019\t\"Howard County, NE\"\t31093\n\"Buffalo County, NE\"\t31019\t\"Kearney County, NE\"\t31099\n\"Buffalo County, NE\"\t31019\t\"Phelps County, NE\"\t31137\n\"Buffalo County, NE\"\t31019\t\"Sherman County, NE\"\t31163\n\"Burt County, NE\"\t31021\t\"Harrison County, IA\"\t19085\n\"Burt County, NE\"\t31021\t\"Monona County, IA\"\t19133\n\"Burt County, NE\"\t31021\t\"Burt County, NE\"\t31021\n\"Burt County, NE\"\t31021\t\"Cuming County, NE\"\t31039\n\"Burt County, NE\"\t31021\t\"Dodge County, NE\"\t31053\n\"Burt County, NE\"\t31021\t\"Thurston County, NE\"\t31173\n\"Burt County, NE\"\t31021\t\"Washington County, NE\"\t31177\n\"Butler County, NE\"\t31023\t\"Butler County, NE\"\t31023\n\"Butler County, NE\"\t31023\t\"Colfax County, NE\"\t31037\n\"Butler County, NE\"\t31023\t\"Dodge County, NE\"\t31053\n\"Butler County, NE\"\t31023\t\"Lancaster County, NE\"\t31109\n\"Butler County, NE\"\t31023\t\"Platte County, NE\"\t31141\n\"Butler County, NE\"\t31023\t\"Polk County, NE\"\t31143\n\"Butler County, NE\"\t31023\t\"Saunders County, NE\"\t31155\n\"Butler County, NE\"\t31023\t\"Seward County, NE\"\t31159\n\"Butler County, NE\"\t31023\t\"York County, NE\"\t31185\n\"Cass County, NE\"\t31025\t\"Fremont County, IA\"\t19071\n\"Cass County, NE\"\t31025\t\"Mills County, IA\"\t19129\n\"Cass County, NE\"\t31025\t\"Cass County, NE\"\t31025\n\"Cass County, NE\"\t31025\t\"Lancaster County, NE\"\t31109\n\"Cass County, NE\"\t31025\t\"Otoe County, NE\"\t31131\n\"Cass County, NE\"\t31025\t\"Sarpy County, NE\"\t31153\n\"Cass County, NE\"\t31025\t\"Saunders County, NE\"\t31155\n\"Cedar County, NE\"\t31027\t\"Cedar County, NE\"\t31027\n\"Cedar County, NE\"\t31027\t\"Dixon County, NE\"\t31051\n\"Cedar County, NE\"\t31027\t\"Knox County, NE\"\t31107\n\"Cedar County, NE\"\t31027\t\"Pierce County, NE\"\t31139\n\"Cedar County, NE\"\t31027\t\"Wayne County, NE\"\t31179\n\"Cedar County, NE\"\t31027\t\"Clay County, SD\"\t46027\n\"Cedar County, NE\"\t31027\t\"Yankton County, SD\"\t46135\n\"Chase County, NE\"\t31029\t\"Phillips County, CO\"\t08095\n\"Chase County, NE\"\t31029\t\"Yuma County, CO\"\t08125\n\"Chase County, NE\"\t31029\t\"Chase County, NE\"\t31029\n\"Chase County, NE\"\t31029\t\"Dundy County, NE\"\t31057\n\"Chase County, NE\"\t31029\t\"Hayes County, NE\"\t31085\n\"Chase County, NE\"\t31029\t\"Perkins County, NE\"\t31135\n\"Cherry County, NE\"\t31031\t\"Blaine County, NE\"\t31009\n\"Cherry County, NE\"\t31031\t\"Brown County, NE\"\t31017\n\"Cherry County, NE\"\t31031\t\"Cherry County, NE\"\t31031\n\"Cherry County, NE\"\t31031\t\"Grant County, NE\"\t31075\n\"Cherry County, NE\"\t31031\t\"Hooker County, NE\"\t31091\n\"Cherry County, NE\"\t31031\t\"Keya Paha County, NE\"\t31103\n\"Cherry County, NE\"\t31031\t\"Sheridan County, NE\"\t31161\n\"Cherry County, NE\"\t31031\t\"Thomas County, NE\"\t31171\n\"Cherry County, NE\"\t31031\t\"Bennett County, SD\"\t46007\n\"Cherry County, NE\"\t31031\t\"Shannon County, SD\"\t46113\n\"Cherry County, NE\"\t31031\t\"Todd County, SD\"\t46121\n\"Cherry County, NE\"\t31031\t\"Tripp County, SD\"\t46123\n\"Cheyenne County, NE\"\t31033\t\"Logan County, CO\"\t08075\n\"Cheyenne County, NE\"\t31033\t\"Sedgwick County, CO\"\t08115\n\"Cheyenne County, NE\"\t31033\t\"Banner County, NE\"\t31007\n\"Cheyenne County, NE\"\t31033\t\"Cheyenne County, NE\"\t31033\n\"Cheyenne County, NE\"\t31033\t\"Deuel County, NE\"\t31049\n\"Cheyenne County, NE\"\t31033\t\"Garden County, NE\"\t31069\n\"Cheyenne County, NE\"\t31033\t\"Kimball County, NE\"\t31105\n\"Cheyenne County, NE\"\t31033\t\"Morrill County, NE\"\t31123\n\"Clay County, NE\"\t31035\t\"Adams County, NE\"\t31001\n\"Clay County, NE\"\t31035\t\"Clay County, NE\"\t31035\n\"Clay County, NE\"\t31035\t\"Fillmore County, NE\"\t31059\n\"Clay County, NE\"\t31035\t\"Hamilton County, NE\"\t31081\n\"Clay County, NE\"\t31035\t\"Nuckolls County, NE\"\t31129\n\"Clay County, NE\"\t31035\t\"Webster County, NE\"\t31181\n\"Clay County, NE\"\t31035\t\"York County, NE\"\t31185\n\"Colfax County, NE\"\t31037\t\"Butler County, NE\"\t31023\n\"Colfax County, NE\"\t31037\t\"Colfax County, NE\"\t31037\n\"Colfax County, NE\"\t31037\t\"Cuming County, NE\"\t31039\n\"Colfax County, NE\"\t31037\t\"Dodge County, NE\"\t31053\n\"Colfax County, NE\"\t31037\t\"Platte County, NE\"\t31141\n\"Colfax County, NE\"\t31037\t\"Stanton County, NE\"\t31167\n\"Cuming County, NE\"\t31039\t\"Burt County, NE\"\t31021\n\"Cuming County, NE\"\t31039\t\"Colfax County, NE\"\t31037\n\"Cuming County, NE\"\t31039\t\"Cuming County, NE\"\t31039\n\"Cuming County, NE\"\t31039\t\"Dodge County, NE\"\t31053\n\"Cuming County, NE\"\t31039\t\"Stanton County, NE\"\t31167\n\"Cuming County, NE\"\t31039\t\"Thurston County, NE\"\t31173\n\"Cuming County, NE\"\t31039\t\"Wayne County, NE\"\t31179\n\"Custer County, NE\"\t31041\t\"Blaine County, NE\"\t31009\n\"Custer County, NE\"\t31041\t\"Buffalo County, NE\"\t31019\n\"Custer County, NE\"\t31041\t\"Custer County, NE\"\t31041\n\"Custer County, NE\"\t31041\t\"Dawson County, NE\"\t31047\n\"Custer County, NE\"\t31041\t\"Garfield County, NE\"\t31071\n\"Custer County, NE\"\t31041\t\"Lincoln County, NE\"\t31111\n\"Custer County, NE\"\t31041\t\"Logan County, NE\"\t31113\n\"Custer County, NE\"\t31041\t\"Loup County, NE\"\t31115\n\"Custer County, NE\"\t31041\t\"Sherman County, NE\"\t31163\n\"Custer County, NE\"\t31041\t\"Valley County, NE\"\t31175\n\"Dakota County, NE\"\t31043\t\"Woodbury County, IA\"\t19193\n\"Dakota County, NE\"\t31043\t\"Dakota County, NE\"\t31043\n\"Dakota County, NE\"\t31043\t\"Dixon County, NE\"\t31051\n\"Dakota County, NE\"\t31043\t\"Thurston County, NE\"\t31173\n\"Dakota County, NE\"\t31043\t\"Union County, SD\"\t46127\n\"Dawes County, NE\"\t31045\t\"Box Butte County, NE\"\t31013\n\"Dawes County, NE\"\t31045\t\"Dawes County, NE\"\t31045\n\"Dawes County, NE\"\t31045\t\"Sheridan County, NE\"\t31161\n\"Dawes County, NE\"\t31045\t\"Sioux County, NE\"\t31165\n\"Dawes County, NE\"\t31045\t\"Fall River County, SD\"\t46047\n\"Dawes County, NE\"\t31045\t\"Shannon County, SD\"\t46113\n\"Dawson County, NE\"\t31047\t\"Buffalo County, NE\"\t31019\n\"Dawson County, NE\"\t31047\t\"Custer County, NE\"\t31041\n\"Dawson County, NE\"\t31047\t\"Dawson County, NE\"\t31047\n\"Dawson County, NE\"\t31047\t\"Frontier County, NE\"\t31063\n\"Dawson County, NE\"\t31047\t\"Gosper County, NE\"\t31073\n\"Dawson County, NE\"\t31047\t\"Lincoln County, NE\"\t31111\n\"Dawson County, NE\"\t31047\t\"Phelps County, NE\"\t31137\n\"Deuel County, NE\"\t31049\t\"Sedgwick County, CO\"\t08115\n\"Deuel County, NE\"\t31049\t\"Cheyenne County, NE\"\t31033\n\"Deuel County, NE\"\t31049\t\"Deuel County, NE\"\t31049\n\"Deuel County, NE\"\t31049\t\"Garden County, NE\"\t31069\n
